vi "Save Transport ITX File.vi"(8 "error in (no error)":errorcluster, 9 "Wavenames":string[](array[string]), 10 "Data":cluster{"Decimated and Filtered Array":dbl[]}[](array[cluster]), 11 "Control Experiment in":refnum<class "Control Experiment.lvclass">) -> (0 "error out":errorcluster, 3 "Control Experiment out":refnum<class "Control Experiment.lvclass">)   [LabVIEW 2016, in "Control Experiment.lvclass"]
uses:
  Control Experiment.lvclass
  <userlib>/_MGI/File/MGI Create Directory Chain Behavior Enum.ctl
  Control Experiment.lvclass/Control Experiment.ctl
  <userlib>/LevyLab/LV to ITX/LVtoITX.lvclass
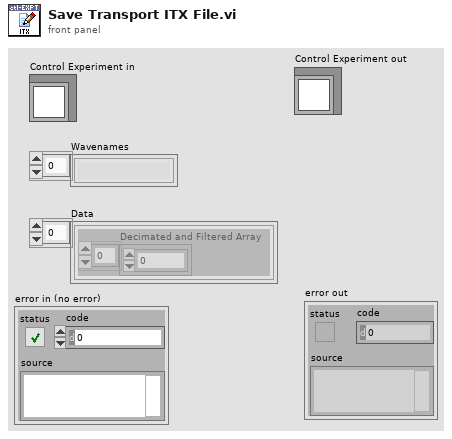
[diagram p1: front panel]
types:
  T1 = typedef "MGI Create Directory Chain Behavior Enum.ctl" = enum16{"Auto Detect", "Path Contains a File", "Path Does Not Contain a File"}
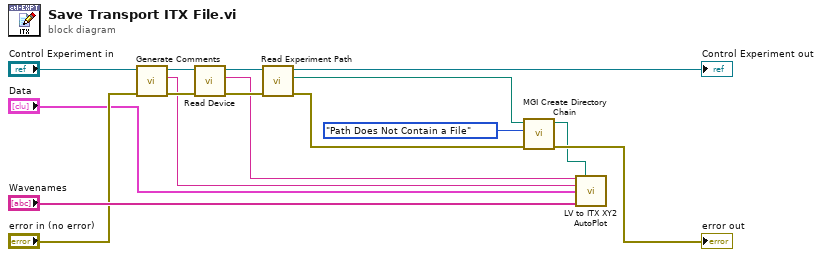
[diagram p0: block diagram]
diagram:
  n1 = call "Generate Comments.vi"("error in (no error)"="error in (no error)", "Control Experiment"="Control Experiment in") -> ("error out"=w12:errorcluster, "Comments"=w7:string, "Control Experiment out"=w16:refnum<class "Control Experiment.lvclass">)  [unwired: 6 in]
  n2 = call "Read Device.vi"("error in (no error)"=w12, "Control Experiment in"=w16) -> ("error out"=w11:errorcluster, "Device"=w6:string, "Control Experiment out"=w14:refnum<class "Control Experiment.lvclass">)  [unwired: 7 in]
  n3 = call "Read Experiment Path.vi"("error in (no error)"=w11, "Control Experiment in"=w14) -> ("error out"=w4:errorcluster, "Experiment Path"=w1:path, "Control Experiment out"=→"Control Experiment out":refnum<class "Control Experiment.lvclass">)  [unwired: 7 in]
  n4 = call <userlib>:"MGI Create Directory Chain.vi"("Error In"=w4, "File Presence (Auto Detect)"=MGI_Create_Directory_Chain_Behavior_Enum."Path Does Not Contain a File", "Path"=w1) -> ("Error Out"=→"error out":errorcluster, "Duplicate Path"=w2:path)  [unwired: 7 in]
  n5 = call <userlib>:"LV to ITX XY2 AutoPlot.vi"("filename"=w6, "path"=w2, "Notes"=w7, "Data"="Data", "wavenames (.Vx, etc)"="Wavenames") -> ()  [unwired: 10 in, 1 out]
